vi "PrintLabel v0.4.vi"(10 "PrintPara":string[](array[string])) -> (0 "error out":errorcluster)   [LabVIEW 2017]
doc: "v0.5:\nAdded reading VISA resource name from a txt file\n\nv0.4:\nAdded reading from text file option\nadded path as an input"
uses:
  <vilib>/Instr/_visa.llb/VISA Configure Serial Port (Instr).vi
panel:
  in  "End Write on Termination Character?":bool=TRUE
  in  "VISA resource name 2":refnum<visa-resource-name>="COM1"
  out "FileFound?":bool
  out "OutputString":string
  in  "write buffer":string="\u0010CT~~CD,~CC^~CT~\n^XA~TA000~JSB^LT12^MNW^MTT^PON^PMN^LH0,0^JMA^PR2,2~SD20^JUS^LRN^CI0^XZ\n~DG000.GRF,01536,016,\n,:::::::::::::::::::::::Q0240,P01240,O0H1B48,O08C809,O040H0B,O070302,N0203FF040,N01C7FF880,P0IFC80,N0H1IFE30,N073FHFE60,O03FIF40,N073FIF3808F3F92044BDE0,N047FIF600C924770648920,V01C824650A48920,N040I03401E9646F0F49920,O080H034032F6469H9799E0,O080H0340,O01800840,R01830,N031C0H030,O0628A380,O020720,O018703,O084860,O084810,P0H4D0,,P04018,Q03,,:::O03E0J03E8040,O012001004D8040,O03FEDAFE175DA0,O031345583ADB60,M0142145FEC2B5BAA88,,::::::::::::::::::::::::::::::::~DG001.GRF,00768,008,\n,::::::::::::::::::::::K01FF80,K0C0070,J031FF0C,J0CFC3E2,I013399E980,I027799E640,I058399C920,I0B81C39H90,H017C4FF99D0,H027E70083E8,H021E4F827E4,H052737C1FD4,H0542FBE080A,H0B19FDE04DA,H0BE5FHF0218,H03C87FF033D,017FJFH07D,017F7FHF81FD,:017F7FHF80FC,017F03FF80FC,017F01F980FC,017F00F181FC,017F00F181FD,017F00FFA1FD,017FBFIF9FD,H0BF9FIFBFD,H0BFCE0033F8,H0BFC0I07FA,H05FE0I0HF2,H05FF0H01FF4,H02FEC0061E4,H027C701C9E8,H01396FFCCD0,I0904D04DB0,I04E498E120,I026C9CFCC0,I013C9EF9,J0CE3E62,J030FF08,K0E0060,K01FF,,::::::::::::::::::::::::::::::~DG002.GRF,01536,048,\n,:::::H070H0H620M070I020J07FC0K0180J040J038001FFC0O0318C003FE0H0400C00800C,H070H0I6N070I060J07FE0K0180J0C0J07C001FFC0O06186003FF0H0C00C01800C,H0D8006060M0D80H060J06060K0180J0C0J0HEH0180Q06186003030H0C00C01800C,H0D8006060M0D80H060J06030K0180J0C0J0C600180Q0C18300301800C00C01800C,:01DC0F66FB063E001DC306F83800603360E03D9830F1F0F0H0C6001800CE07B0F600C18300301B07F00C03E1EC,018C1FE6FB067F0018C306F8FE006033F3F87F9831F9F1F8004C001800FF0FF1FE00C18300301B07F00C03E3FC,018C18E6618CE38018C30660C600603383186398319CC31C0078001800E38C718E01818180301904C00C01831C,018C30E6618CC18018C30661C7006063071CC398330CC30C0070H01FF8C19C738E0181818030318CC00C01861C,0306306H618C01803063066183007FE3060CC1983300C30I0F8001FF8C1983306018181803FF18CC00C01860C,0306306H60D807803063066183007F83060CC1983300C3C00199801800C1983306018181803FC18CC00C01860C,03FE306H60D83D803FE3066183006003060CC1983300C1F8030D801800C19833060181818030018CC00C01860C,03FE306H60D861803FE3066183006003060CC1983300C03C0307001800C19833060181818030H0D8C00C01860C,0603306H60D8C1806033066183006003060CC198330CC00C0307001800C19833060181818030H0D8C00C01860C,0603386H6070C38060330661C7006003071CE198330CC30C0307001800C19833060181818030H0D8C00C01870C,060318E66070E38060338E60C60060030318639C7198C38C018F801800C18C718E0181818030H0D8C00C01831C,0C019FE678707D80C019F678FE00600303F87F8FB1F8F1F801FCC01FFCC18FF1FE00C1830030H070F00FF9E3FC,0C01876638603980C018E6383800600300E01D8730F070F0H0F8801FFCC187B0F600C1830030H070700FF8E0EC,P060hP0300600C003,P060hN018330600C003,P0C0hN01C638C006006,O01C0hO0FE1FC006006,O0180hO07C0F800300C,,::~DG003.GRF,01536,024,\n,:::::::::::::::::::::::::::::::3F80M0H1H0430I03E0I020K081FC3F82,2040M02180C40I0410I020J0141022041,2020M02180C40I08080H020J0141012021,202412F070021414F1D010H0703A1C100221012021,20241308H8041414423010H0H846220H0H2101202080,2044120904041224H41010010482410H0H2102204080,3F84120904041224H41010010482410H0411FC3F8080,20041209FC04124I410100104827F0H07F10020H080,200412090H04114I4101001048240I08090020H080,200412090404114I41008090482410H08090020H080,20043208H8041084423004108846220010050020H080,2003D2087002108441D003E0703A1C101005002001,Q020K010gG01,Q020J0420gG01,Q010J03C0gG02,,::::::::::::::::^XA\n^MMT\n^PW446\n^LL0219\n^LS0\n^FT0,96^XG000.GRF,1,1^FS\n^FT352,96^XG001.GRF,1,1^FS\n^FT32,96^XG002.GRF,1,1^FS\n^FT128,128^XG003.GRF,1,1^FS\n^FO25,18^GB382,183,4^FS\n^FO29,65^GB376,0,1^FS\n^FT104,132^A@N,17,18,TT0003M_^FH\\^CI17^F8^FDPart No :^FS^CI0\n^FT62,163^A@N,17,18,TT0003M_^FH\\^CI17^F8^FDDescription :^FS^CI0\n^FT181,137^A0N,28,28^FH\\^FD5EF.839.461^FS\n^FT167,170^A0N,28,28^FH\\^FDRear Power LH^FS\n^FT40,190^A@N,14,13,TT0003M_^FH\\^CI17^F8^FDID:^FS^CI0\n^FT63,192^A0N,17,16^FH\\^FDXX^FS\n^FT175,189^A@N,14,13,TT0003M_^FH\\^CI17^F8^FDDATE:^FS^CI0\n^FT217,191^A0N,17,16^FH\\^FD241213-1538^FS\n^PQ1,0,1,Y^XZ\n^XA^ID000.GRF^FS^XZ\n^XA^ID001.GRF^FS^XZ\n^XA^ID002.GRF^FS^XZ\n^XA^ID003.GRF^FS^XZ\n"
  # "~TA000 ===> How much label should come out by. 080->1cm."
  # "0- <Name in ini>\n1- <Common Name>\n \n2- Part No\n3- Name\n4- ID\n5- DATE-Time\n6- Count"
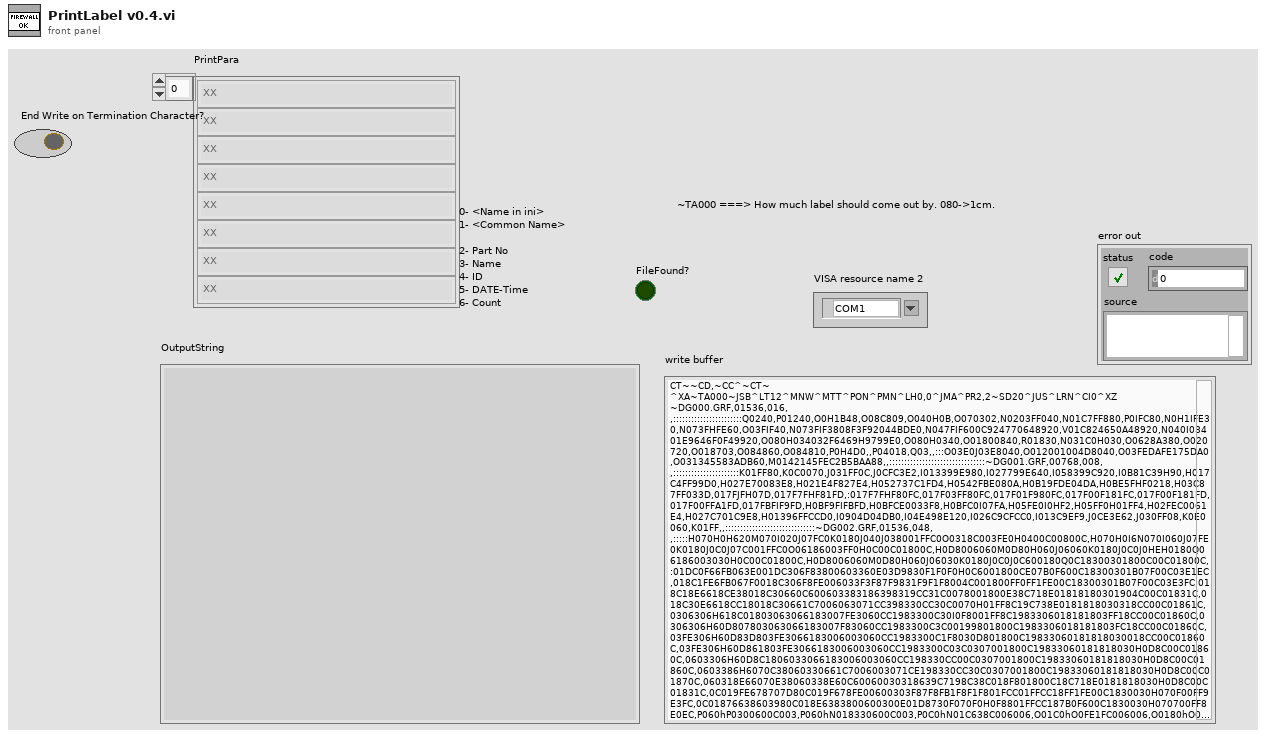
[diagram p1: front panel]
types:
  T1 = cluster{"XON":enum16{"NUL", "SOH", "STX", "ETX", "EOT", "ENQ", "ACK", "BEL", "BS", "HT", "LF", "VT", "FF", "CR", "SO", "SI", "DLE", "DC1", "DC2", "DC3", "DC4", "NAK", "SYN", "ETB", "CAN", "EM", "SUB", "ESC", "FS", "GS", "RS", "US", "SP", "!", "\"", "#", "$", "%", "&", "'", "(", ")", "*", "+", ",", "- (-)", ".", "/", "0", "1", "2", "3", "4", "5", "6", "7", "8", "9", ":", ";", "<", "=", ">", "?", "@", "A", "B", "C", "D", "E", "F", "G", "H", "I", "J", "K", "L", "M", "N", "O", "P", "Q", "R", "S", "T", "U", "V", "W", "X", "Y", "Z", "[", "\\", "]", "^", "_", "`", "a", "b", "c", "d", "e", "f", "g", "h", "i", "j", "k", "l", "m", "n", "o", "p", "q", "r", "s", "t", "u", "v", "w", "x", "y", "z", "{", "|", "}", "~"}, "XOFF":enum16{"NUL", "SOH", "STX", "ETX", "EOT", "ENQ", "ACK", "BEL", "BS", "HT", "LF", "VT", "FF", "CR", "SO", "SI", "DLE", "DC1", "DC2", "DC3", "DC4", "NAK", "SYN", "ETB", "CAN", "EM", "SUB", "ESC", "FS", "GS", "RS", "US", "SP", "!", "\"", "#", "$", "%", "&", "'", "(", ")", "*", "+", ",", "- (-)", ".", "/", "0", "1", "2", "3", "4", "5", "6", "7", "8", "9", ":", ";", "<", "=", ">", "?", "@", "A", "B", "C", "D", "E", "F", "G", "H", "I", "J", "K", "L", "M", "N", "O", "P", "Q", "R", "S", "T", "U", "V", "W", "X", "Y", "Z", "[", "\\", "]", "^", "_", "`", "a", "b", "c", "d", "e", "f", "g", "h", "i", "j", "k", "l", "m", "n", "o", "p", "q", "r", "s", "t", "u", "v", "w", "x", "y", "z", "{", "|", "}", "~"}}
  T2 = cluster{"baud rate":u32, "data bits":u16, "parity":enum16{"None", "Odd", "Even", "Mark", "Space"}, "stop bits":u16, "flow control":u16}
  T3 = enum16{"NUL", "SOH", "STX", "ETX", "EOT", "ENQ", "ACK", "BEL", "BS", "HT", "LF", "VT", "FF", "CR", "SO", "SI", "DLE", "DC1", "DC2", "DC3", "DC4", "NAK", "SYN", "ETB", "CAN", "EM", "SUB", "ESC", "FS", "GS", "RS", "US", "SP", "!", "\"", "#", "$", "%", "&", "'", "(", ")", "*", "+", ",", "- (-)", ".", "/", "0", "1", "2", "3", "4", "5", "6", "7", "8", "9", ":", ";", "<", "=", ">", "?", "@", "A", "B", "C", "D", "E", "F", "G", "H", "I", "J", "K", "L", "M", "N", "O", "P", "Q", "R", "S", "T", "U", "V", "W", "X", "Y", "Z", "[", "\\", "]", "^", "_", "`", "a", "b", "c", "d", "e", "f", "g", "h", "i", "j", "k", "l", "m", "n", "o", "p", "q", "r", "s", "t", "u", "v", "w", "x", "y", "z", "{", "|", "}", "~"}
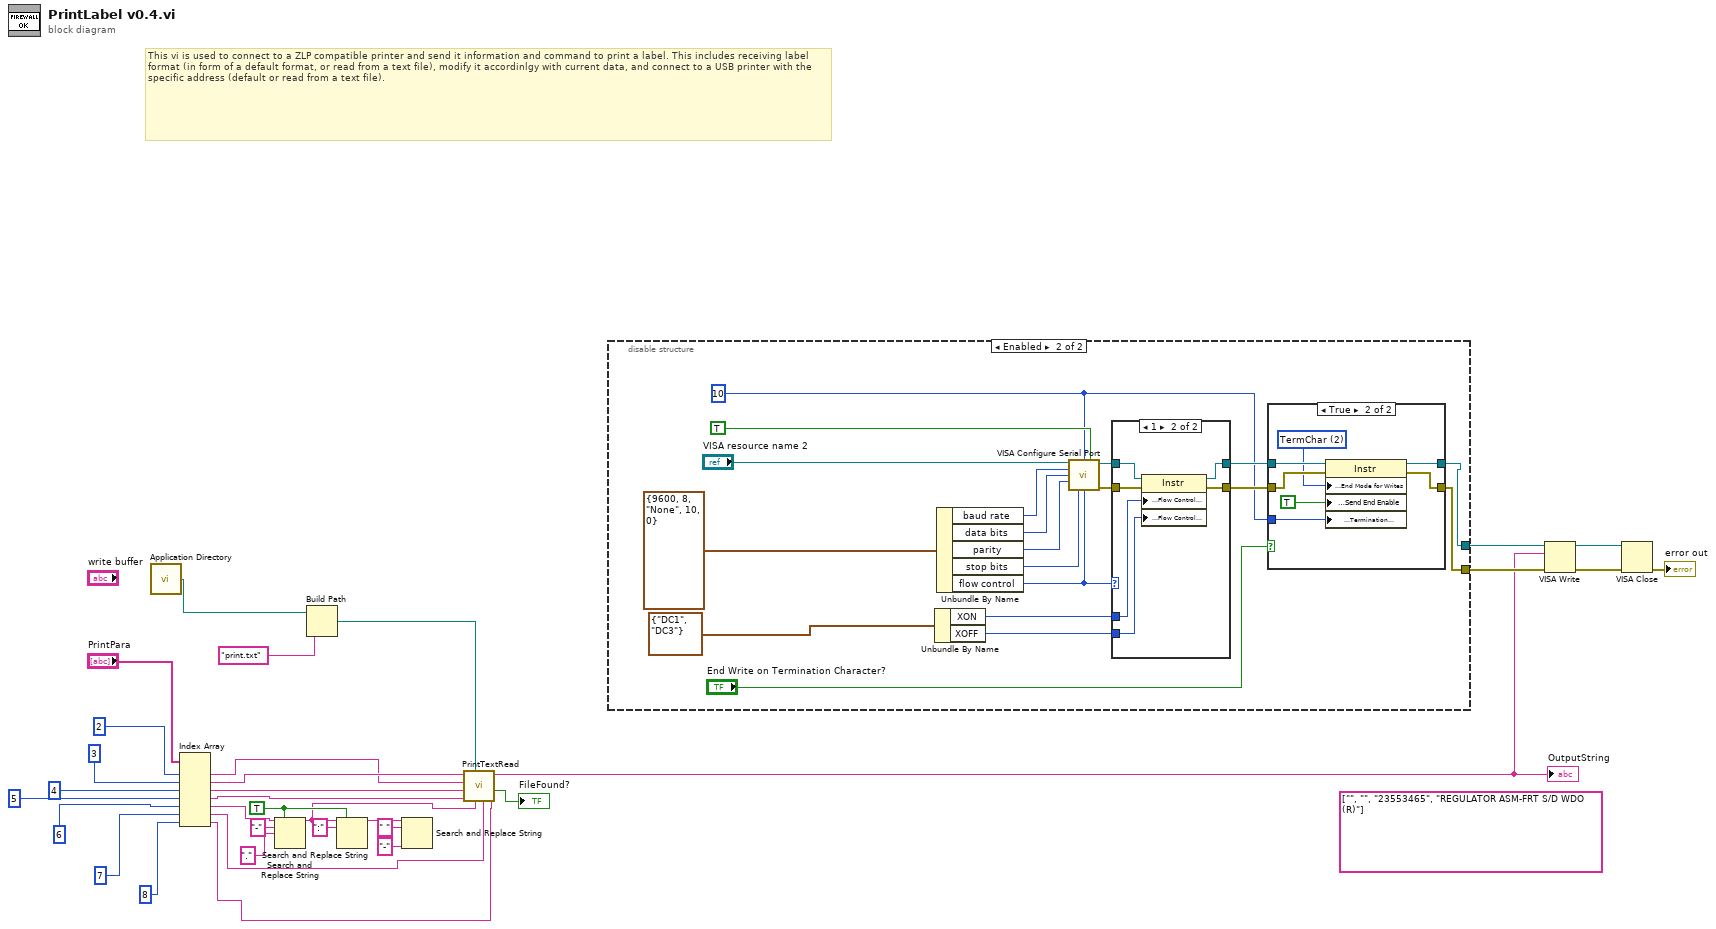
[diagram p0: block diagram]
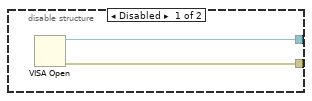
[diagram p2: hidden frame]
diagram:
  (unwired) string[] ["", "", "23553465", "REGULATOR ASM-FRT S/D WDO (R)"] ("PrintPara")
  w17 = TRUE ("replace all? (F)")
  # "This vi is used to connect to a ZLP compatible printer and send it information and command to print a label. This includes receiving label format (in form of a default format, or read from a text file), modify it accordinlgy with current data, and connect to a USB printer with the specific address (default or read from a text file)."
  n1 = call <vilib>:"Application Directory.vi"() -> ("Application Directory"=w13:path)
  n2 = Index Array(array="PrintPara", index #1=2 ("index"), index #2=3 ("index"), index #3=4 ("index"), index #4=5 ("index"), index #5=6 ("index"), index #6=7 ("index"), index #7=8 ("index")) -> (element #1=w11:string, element #2=w12:string, element #3=w21:string, element #4=w5:string, element #5=w4:string, element #6=w2:string, element #7=w1:string)
  n3 = Search and Replace String(replace all?=w17, input string=w4, search string="-" ("regular expression (\"\")"), replace string="." ("replace string (\"\")")) -> (result string=w3:string)  [unwired: 4 in, 3 out]
  n4 = Build Path(base path=w13, name or relative path="print.txt") -> (appended path=w22:path)
  n5 = Search and Replace String(replace all?=w17, input string=w3, search string=":" ("regular expression (\"\")")) -> (result string=w16:string)  [unwired: 5 in, 3 out]
  n6 = Search and Replace String(input string=w16, search string=" ", replace string="-" ("replace string (\"\")")) -> ()  [unwired: 5 in, 4 out]
  n7 = call "PrintTextRead.vi"("No"=w1, "Time"=w2, "Date"=w3, "file path (use dialog)"=w22, "Shift"=w5, "ID"=w21, "PartNumber"=w11, "Description"=w12) -> ("FileFound?"=→"FileFound?":bool, "result string"=w20:string)  [unwired: 2 in]
  "OutputString" <- w20
  n8 = disable-structure shown="Enabled" {
    disable-tunnel: [w36 w37] -> w33
    disable-tunnel: [w35 w38] -> w32
    frame Disabled {
      n9 = VISA Open() -> (VISA resource name=w35:refnum<visa-resource-name>, VISA resource name=w34:refnum<visa-resource-name>, error out=w36:errorcluster)  [unwired: 4 in]
    }
    frame Enabled {
      w39 = u8 10 ("Termination Character")
      n10 = Unbundle By Name(T1 {"XON"=enum."DC1", "XOFF"=enum."DC3"} ("XON/XOFF Characters")) -> ("XON"=w44:T3, "XOFF"=w43:T3)
      n11 = Unbundle By Name(T2 {"baud rate"=9600, "data bits"=8, "parity"=enum."None", "stop bits"=10, "flow control"=0} ("Serial Settings")) -> ("baud rate"=w48:u32, "data bits"=w49:u16, "parity"=w50:enum16{"None", "Odd", "Even", "Mark", "Space"}, "stop bits"=w51:u16, "flow control"=w45:u16)
      n12 = call-poly "VISA Configure Serial Port"("VISA resource name"="VISA resource name 2", "termination char\n(0xA = '\\n' = LF)"=w39, "Enable Termination\nChar (T)"=TRUE ("End Read on Termination Character?"), "baud rate (9600)"=w48, "data bits (8)"=w49, "parity (0:none)"=w50, "stop bits (10: 1 bit)"=w51, "flow control (0:none)"=w45) -> ("VISA resource name out"=w52:refnum<visa-resource-name>, "error out"=w53:errorcluster)  [unwired: 2 in, 4 out]
      n13 = case shown="1" w45 {
        tunnel: [w65 w72] -> w42
        tunnel: [w66 w71] -> w41
        tunnel: w53 -> [w65 w70]
        tunnel: w52 -> [w66 w69]
        tunnel: w44 -> [_ w68]
        tunnel: w43 -> [_ w67]
        frame Default {
        }
        frame 1 {
          n14 = property class="Instr"(reference=w69, error in=w70, "Serial Settings:Flow Control XON Character"=w68, "Serial Settings:Flow Control XOFF Character"=w67) -> (reference out=w71:refnum<visa-resource-name>, error out=w72:errorcluster)
        }
      }
      n15 = case shown="True" "End Write on Termination Character?" {
        tunnel: w41 -> [w56 w64]
        tunnel: w42 -> [w57 w63]
        tunnel: [w56 w62] -> w38
        tunnel: [w57 w61] -> w37
        tunnel: w39 -> [_ w59]
        frame False {
        }
        frame True {
          w60 = u16 2 items=["None", "LastBit", "TermChar", "Break"] ("Serial Settings:Serial End Mode for Writes")
          n16 = property class="Instr"(reference=w64, error in=w63, "Serial Settings:End Mode for Writes"=w60, "Message Based Settings:Send End Enable"=TRUE, "Message Based Settings:Termination Character"=w59) -> (reference out=w62:refnum<visa-resource-name>, error out=w61:errorcluster)
        }
      }
    }
  }
  n17 = VISA Write(VISA resource name=w32, write buffer=w20, error in (no error)=w33) -> (VISA resource name out=w30:refnum<visa-resource-name>, error out=w31:errorcluster)  [unwired: 1 out]
  n18 = VISA Close(VISA resource name=w30, error in (no error)=w31) -> (error out=→"error out":errorcluster)
